vi "_appendImage.vi"(8 "error in (no error)":errorcluster, 10 "Image Path":path) -> (0 "error out":errorcluster)   [LabVIEW 2017]
uses:
  Support/File Stream/File Stream.lvlib
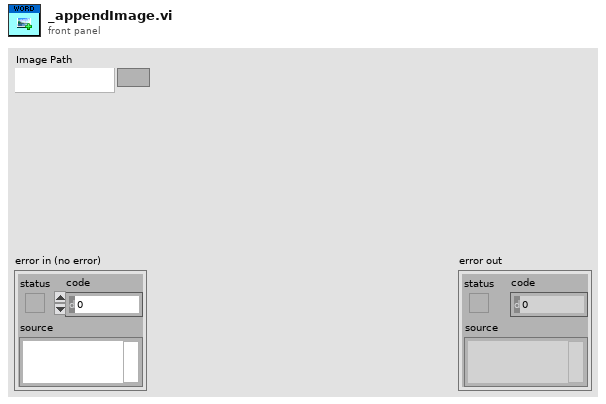
[diagram p1: front panel]
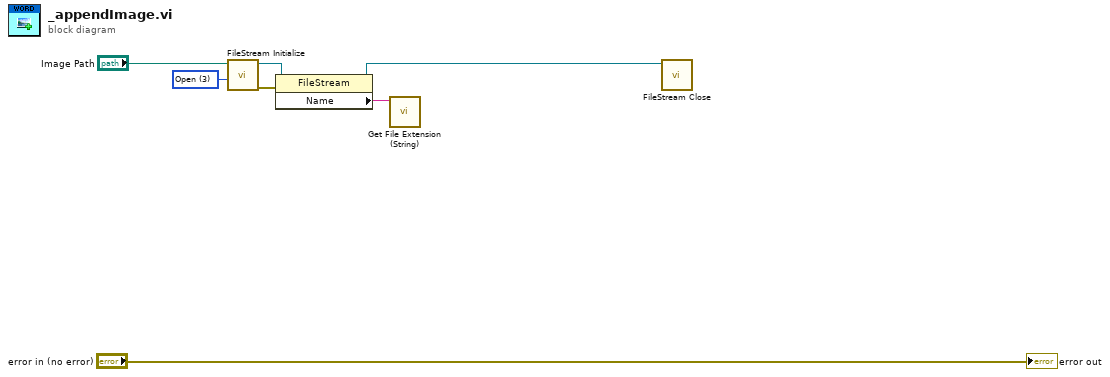
[diagram p0: block diagram]
diagram:
  w4 = 3 items=["CreateNew"=1, "Create"=2, "Open"=3, "OpenOrCreate"=4, "Truncate"=5, "Append"=6] ("mode")
  n1 = call "FileStream Initialize.vi"("mode"=w4, "path"="Image Path") -> ("error out"=w2:errorcluster, "new reference"=w5:refnum<k24>)  [unwired: 8 in]
  n2 = property class="FileStream"(reference=w5, error in=w2) -> (reference out=w3:refnum<k24>, "Name"=w1:string)  [unwired: 1 out]
  n3 = call "Get File Extension (String).vi"("File Path"=w1) -> ()  [unwired: 9 in, 2 out]
  n4 = call "FileStream Close.vi"("reference"=w3) -> ()  [unwired: 10 in, 1 out]
  "error out" <- "error in (no error)"
